vi "AppData - Handle.vi"(4 "error in":errorcluster, 6 "Action":T2, 7 "Data In":T1 {"LogStartTime" format="%<%x %.3X>T"}) -> (0 "error out":errorcluster, 3 "Data Out":T1 {"LogStartTime" format="%<%x %.3X>T"})   [LabVIEW 2023]
uses:
  controls/Action Enum.ctl
  controls/UI Data.ctl
  <vilib>/NI/Modbus Library/API/Master/Modbus Master.lvclass
  LibreVNA/LibreVNA.lvclass
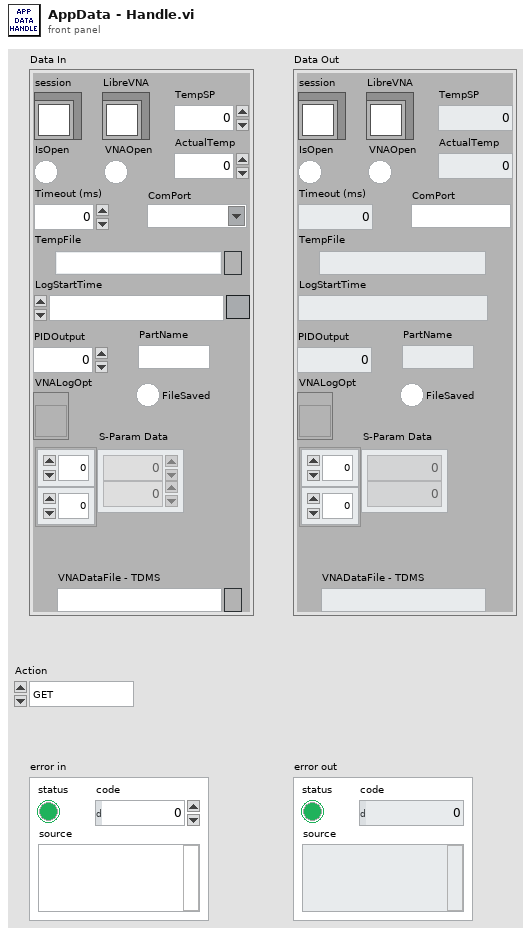
[diagram p1: front panel]
types:
  T1 = typedef "UI Data.ctl" = cluster{"session":refnum<class "Modbus Master.lvclass">, "IsOpen":bool, "Timeout (ms)":i32, "TempFile":path, "LogStartTime":timestamp, "LibreVNA":refnum<class "LibreVNA.lvclass">, "VNAOpen":bool, "TempSP":dbl, "ActualTemp":dbl, "FileSaved":bool, "PIDOutput":dbl, "VNALogOpt":refnum<vi>, "PartName":string, "ComPort":refnum<visa-resource-name>, "S-Param Data":dbl[][], "VNADataFile - TDMS":path}
  T2 = typedef "Action Enum.ctl" = enum16{"GET", "SET", "RESET"}
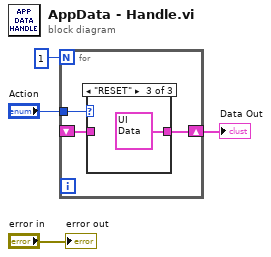
[diagram p0: block diagram]
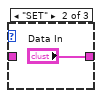
[diagram p3: hidden frame]
diagram:
  n1 = for {
    N: 1 -> [_]
    tunnel: "Action" -> [w7]
    shift-right: [w6] -> w2
    shift-left: _ -> [w5]
    n2 = case shown="\"RESET\"" w7 {
      tunnel: [w8 "Data In" T1 {"session"=refnum, "IsOpen"=FALSE, "Timeout (ms)"=0, "TempFile"=path "", "LogStartTime"=timestamp(0 s since 1904-01-01), "LibreVNA"=refnum, "VNAOpen"=FALSE, "TempSP"=0.0, "ActualTemp"=0.0, "FileSaved"=FALSE, "PIDOutput"=0.0, "VNALogOpt"=refnum, "PartName"="", "ComPort"="", "S-Param Data"=[], "VNADataFile - TDMS"=path ""} ("Data In")] -> w6
      tunnel: w5 -> [w8 _ _]
      frame "GET", Default {
      }
      frame "SET" {
      }
      frame "RESET" {
      }
    }
  }
  "Data Out" <- w2
  "error out" <- "error in"
